vi "rsidr_core_global.vi"() -> ()   [LabVIEW 2015, in "Rohde&Schwarz CMXP NR FR2 Measurement.lvlib"] (continued)
peak values for low and high EVM window position, for all measured list mode segments.\n\nAvailable Repeated Capabilities:\ninstance: i0, i1, i2, i3, i4, i5, i6, i7, i8, i9, i10, i11, i12, i13, i14, i15, i16, i17, i18, i19, i20, i21, i22, i23, i24, i25, i26, i27, i28, i29, i30, i31, i32\r\n\nRemote-control command(s):\nCALCulate:NRMMw:MEAS<i>:MEValuation:LIST:MODulation:PERRor:PEAK:LOW:CURRent?"}, {"Level"=5, "Class Only"=FALSE, "Identifier"="RSCMXPNRFR2M_ATTR_QUERY_MULTI_EVAL_MEASUREMENT_LIST_PERR_PEAK_LOW_EXTREME_LIMIT_CHECK_RESULTS", "Descriptive Name"="Query Multi Eval Measurement List PERR Peak Low Extreme Limit Check Results", "Data Type"=enum."RawString", "Command"="CALC:NRMM:MEAS{instance}:MEV:LIST:MOD:PERR:PEAK:LOW:EXTR?", "Access"=enum."Read Only", "Range Table"="", "Read Callback"="", "Write Callback"="", "Range Callback"="", "Check Callback"="", "Rngtable Callback"="", "Coerce Callback"="", "Supported Models"="", "Instrument Options"="", "Check Status Callback"="", "Flags"=0, "Help"="Returns the limit check results for the phase error peak values for low and high EVM window position, for all measured list mode segments.\n\nAvailable Repeated Capabilities:\ninstance: i0, i1, i2, i3, i4, i5, i6, i7, i8, i9, i10, i11, i12, i13, i14, i15, i16, i17, i18, i19, i20, i21, i22, i23, i24, i25, i26, i27, i28, i29, i30, i31, i32\r\n\nRemote-control command(s):\nCALCulate:NRMMw:MEAS<i>:MEValuation:LIST:MODulation:PERRor:PEAK:LOW:EXTReme?"}, {"Level"=5, "Class Only"=FALSE, "Identifier"="RSCMXPNRFR2M_ATTR_FETCH_MULTI_EVAL_MEASUREMENT_LIST_PERR_RMS_HIGH_AVERAGE_RESULTS", "Descriptive Name"="Fetch Multi Eval Measurement List PERR RMS High Average Results", "Data Type"=enum."RawString", "Command"="FETC:NRMM:MEAS{instance}:MEV:LIST:MOD:PERR:RMS:HIGH:AVER?", "Access"=enum."Read Only", "Range Table"="", "Read Callback"="", "Write Callback"="", "Range Callback"="", "Check Callback"="", "Rngtable Callback"="", "Coerce Callback"="", "Supported Models"="", "Instrument Options"="", "Check Status Callback"="", "Flags"=0, "Help"="Returns phase error RMS values for low and high EVM window position, for all measured list mode segments.\n\nAvailable Repeated Capabilities:\ninstance: i0, i1, i2, i3, i4, i5, i6, i7, i8, i9, i10, i11, i12, i13, i14, i15, i16, i17, i18, i19, i20, i21, i22, i23, i24, i25, i26, i27, i28, i29, i30, i31, i32\r\n\nRemote-control command(s):\nFETCh:NRMMw:MEAS<i>:MEValuation:LIST:MODulation:PERRor:RMS:HIGH:AVERage?"}, {"Level"=5, "Class Only"=FALSE, "Identifier"="RSCMXPNRFR2M_ATTR_FETCH_MULTI_EVAL_MEASUREMENT_LIST_PERR_RMS_HIGH_CURRENT_RESULTS", "Descriptive Name"="Fetch Multi Eval Measurement List PERR RMS High Current Results", "Data Type"=enum."RawString", "Command"="FETC:NRMM:MEAS{instance}:MEV:LIST:MOD:PERR:RMS:HIGH:CURR?", "Access"=enum."Read Only", "Range Table"="", "Read Callback"="", "Write Callback"="", "Range Callback"="", "Check Callback"="", "Rngtable Callback"="", "Coerce Callback"="", "Supported Models"="", "Instrument Options"="", "Check Status Callback"="", "Flags"=0, "Help"="Returns phase error RMS values for low and high EVM window position, for all measured list mode segments.\n\nAvailable Repeated Capabilities:\ninstance: i0, i1, i2, i3, i4, i5, i6, i7, i8, i9, i10, i11, i12, i13, i14, i15, i16, i17, i18, i19, i20, i21, i22, i23, i24, i25, i26, i27, i28, i29, i30, i31, i32\r\n\nRemote-control command(s):\nFETCh:NRMMw:MEAS<i>:MEValuation:LIST:MODulation:PERRor:RMS:HIGH:CURRent?"}, {"Level"=5, "Class Only"=FALSE, "Identifier"="RSCMXPNRFR2M_ATTR_FETCH_MULTI_EVAL_MEASUREMENT_LIST_PERR_RMS_HIGH_EXTREME_RESULTS", "Descriptive Name"="Fetch Multi Eval Measurement List PERR RMS High Extreme Results", "Data Type"=enum."RawString", "Command"="FETC:NRMM:MEAS{instance}:MEV:LIST:MOD:PERR:RMS:HIGH:EXTR?", "Access"=enum."Read Only", "Range Table"="", "Read Callback"="", "Write Callback"="", "Range Callback"="", "Check Callback"="", "Rngtable Callback"="", "Coerce Callback"="", "Supported Models"="", "Instrument Options"="", "Check Status Callback"="", "Flags"=0, "Help"="Returns phase error RMS values for low and high EVM window position, for all measured list mode segments.\n\nAvailable Repeated Capabilities:\ninstance: i0, i1, i2, i3, i4, i5, i6, i7, i8, i9, i10, i11, i12, i13, i14, i15, i16, i17, i18, i19, i20, i21, i22, i23, i24, i25, i26, i27, i28, i29, i30, i31, i32\r\n\nRemote-control command(s):\nFETCh:NRMMw:MEAS<i>:MEValuation:LIST:MODulation:PERRor:RMS:HIGH:EXTReme?"}, {"Level"=5, "Class Only"=FALSE, "Identifier"="RSCMXPNRFR2M_ATTR_FETCH_MULTI_EVAL_MEASUREMENT_LIST_PERR_RMS_HIGH_STANDARD_DEVIATION_RESULTS", "Descriptive Name"="Fetch Multi Eval Measurement List PERR RMS High Standard Deviation Results", "Data Type"=enum."RawString", "Command"="FETC:NRMM:MEAS{instance}:MEV:LIST:MOD:PERR:RMS:HIGH:SDEV?", "Access"=enum."Read Only", "Range Table"="", "Read Callback"="", "Write Callback"="", "Range Callback"="", "Check Callback"="", "Rngtable Callback"="", "Coerce Callback"="", "Supported Models"="", "Instrument Options"="", "Check Status Callback"="", "Flags"=0, "Help"="Returns phase error RMS values for low and high EVM window position, for all measured list mode segments.\n\nAvailable Repeated Capabilities:\ninstance: i0, i1, i2, i3, i4, i5, i6, i7, i8, i9, i10, i11, i12, i13, i14, i15, i16, i17, i18, i19, i20, i21, i22, i23, i24, i25, i26, i27, i28, i29, i30, i31, i32\r\n\nRemote-control command(s):\nFETCh:NRMMw:MEAS<i>:MEValuation:LIST:MODulation:PERRor:RMS:HIGH:SDEViation?"}, {"Level"=5, "Class Only"=FALSE, "Identifier"="RSCMXPNRFR2M_ATTR_FETCH_MULTI_EVAL_MEASUREMENT_LIST_PERR_RMS_LOW_AVERAGE_RESULTS", "Descriptive Name"="Fetch Multi Eval Measurement List PERR RMS Low Average Results", "Data Type"=enum."RawString", "Command"="FETC:NRMM:MEAS{instance}:MEV:LIST:MOD:PERR:RMS:LOW:AVER?", "Access"=enum."Read Only", "Range Table"="", "Read Callback"="", "Write Callback"="", "Range Callback"="", "Check Callback"="", "Rngtable Callback"="", "Coerce Callback"="", "Supported Models"="", "Instrument Options"="", "Check Status Callback"="", "Flags"=0, "Help"="Returns phase error RMS values for low and high EVM window position, for all measured list mode segments.\n\nAvailable Repeated Capabilities:\ninstance: i0, i1, i2, i3, i4, i5, i6, i7, i8, i9, i10, i11, i12, i13, i14, i15, i16, i17, i18, i19, i20, i21, i22, i23, i24, i25, i26, i27, i28, i29, i30, i31, i32\r\n\nRemote-control command(s):\nFETCh:NRMMw:MEAS<i>:MEValuation:LIST:MODulation:PERRor:RMS:LOW:AVERage?"}, {"Level"=5, "Class Only"=FALSE, "Identifier"="RSCMXPNRFR2M_ATTR_FETCH_MULTI_EVAL_MEASUREMENT_LIST_PERR_RMS_LOW_CURRENT_RESULTS", "Descriptive Name"="Fetch Multi Eval Measurement List PERR RMS Low Current Results", "Data Type"=enum."RawString", "Command"="FETC:NRMM:MEAS{instance}:MEV:LIST:MOD:PERR:RMS:LOW:CURR?", "Access"=enum."Read Only", "Range Table"="", "Read Callback"="", "Write Callback"="", "Range Callback"="", "Check Callback"="", "Rngtable Callback"="", "Coerce Callback"="", "Supported Models"="", "Instrument Options"="", "Check Status Callback"="", "Flags"=0, "Help"="Returns phase error RMS values for low and high EVM window position, for all measured list mode segments.\n\nAvailable Repeated Capabilities:\ninstance: i0, i1, i2, i3, i4, i5, i6, i7, i8, i9, i10, i11, i12, i13, i14, i15, i16, i17, i18, i19, i20, i21, i22, i23, i24, i25, i26, i27, i28, i29, i30, i31, i32\r\n\nRemote-control command(s):\nFETCh:NRMMw:MEAS<i>:MEValuation:LIST:MODulation:PERRor:RMS:LOW:CURRent?"}, {"Level"=5, "Class Only"=FALSE, "Identifier"="RSCMXPNRFR2M_ATTR_FETCH_MULTI_EVAL_MEASUREMENT_LIST_PERR_RMS_LOW_EXTREME_RESULTS", "Descriptive Name"="Fetch Multi Eval Measurement List PERR RMS Low Extreme Results", "Data Type"=enum."RawString", "Command"="FETC:NRMM:MEAS{instance}:MEV:LIST:MOD:PERR:RMS:LOW:EXTR?", "Access"=enum."Read Only", "Range Table"="", "Read Callback"="", "Write Callback"="", "Range Callback"="", "Check Callback"="", "Rngtable Callback"="", "Coerce Callback"="", "Supported Models"="", "Instrument Options"="", "Check Status Callback"="", "Flags"=0, "Help"="Returns phase error RMS values for low and high EVM window position, for all measured list mode segments.\n\nAvailable Repeated Capabilities:\ninstance: i0, i1, i2, i3, i4, i5, i6, i7, i8, i9, i10, i11, i12, i13, i14, i15, i16, i17, i18, i19, i20, i21, i22, i23, i24, i25, i26, i27, i28, i29, i30, i31, i32\r\n\nRemote-control command(s):\nFETCh:NRMMw:MEAS<i>:MEValuation:LIST:MODulation:PERRor:RMS:LOW:EXTReme?"}, {"Level"=5, "Class Only"=FALSE, "Identifier"="RSCMXPNRFR2M_ATTR_FETCH_MULTI_EVAL_MEASUREMENT_LIST_PERR_RMS_LOW_STANDARD_DEVIATION_RESULTS", "Descriptive Name"="Fetch Multi Eval Measurement List PERR RMS Low Standard Deviation Results", "Data Type"=enum."RawString", "Command"="FETC:NRMM:MEAS{instance}:MEV:LIST:MOD:PERR:RMS:LOW:SDEV?", "Access"=enum."Read Only", "Range Table"="", "Read Callback"="", "Write Callback"="", "Range Callback"="", "Check Callback"="", "Rngtable Callback"="", "Coerce Callback"="", "Supported Models"="", "Instrument Options"="", "Check Status Callback"="", "Flags"=0, "Help"="Returns phase error RMS values for low and high EVM window position, for all measured list mode segments.\n\nAvailable Repeated Capabilities:\ninstance: i0, i1, i2, i3, i4, i5, i6, i7, i8, i9, i10, i11, i12, i13, i14, i15, i16, i17, i18, i19, i20, i21, i22, i23, i24, i25, i26, i27, i28, i29, i30, i31, i32\r\n\nRemote-control command(s):\nFETCh:NRMMw:MEAS<i>:MEValuation:LIST:MODulation:PERRor:RMS:LOW:SDEViation?"}, {"Level"=5, "Class Only"=FALSE, "Identifier"="RSCMXPNRFR2M_ATTR_QUERY_MULTI_EVAL_MEASUREMENT_LIST_PERR_RMS_HIGH_AVERAGE_LIMIT_CHECK_RESULTS", "Descriptive Name"="Query Multi Eval Measurement List PERR RMS High Average Limit Check Results", "Data Type"=enum."RawString", "Command"="CALC:NRMM:MEAS{instance}:MEV:LIST:MOD:PERR:RMS:HIGH:AVER?", "Access"=enum."Read Only", "Range Table"="", "Read Callback"="", "Write Callback"="", "Range Callback"="", "Check Callback"="", "Rngtable Callback"="", "Coerce Callback"="", "Supported Models"="", "Instrument Options"="", "Check Status Callback"="", "Flags"=0, "Help"="Returns the limit check results for the phase error RMS values for low and high EVM window position, for all measured list mode segments.\n\nAvailable Repeated Capabilities:\ninstance: i0, i1, i2, i3, i4, i5, i6, i7, i8, i9, i10, i11, i12, i13, i14, i15, i16, i17, i18, i19, i20, i21, i22, i23, i24, i25, i26, i27, i28, i29, i30, i31, i32\r\n\nRemote-control command(s):\nCALCulate:NRMMw:MEAS<i>:MEValuation:LIST:MODulation:PERRor:RMS:HIGH:AVERage?"}, {"Level"=5, "Class Only"=FALSE, "Identifier"="RSCMXPNRFR2M_ATTR_QUERY_MULTI_EVAL_MEASUREMENT_LIST_PERR_RMS_HIGH_CURRENT_LIMIT_CHECK_RESULTS", "Descriptive Name"="Query Multi Eval Measurement List PERR RMS High Current Limit Check Results", "Data Type"=enum."RawString", "Command"="CALC:NRMM:MEAS{instance}:MEV:LIST:MOD:PERR:RMS:HIGH:CURR?", "Access"=enum."Read Only", "Range Table"="", "Read Callback"="", "Write Callback"="", "Range Callback"="", "Check Callback"="", "Rngtable Callback"="", "Coerce Callback"="", "Supported Models"="", "Instrument Options"="", "Check Status Callback"="", "Flags"=0, "Help"="Returns the limit check results for the phase error RMS values for low and high EVM window position, for all measured list mode segments.\n\nAvailable Repeated Capabilities:\ninstance: i0, i1, i2, i3, i4, i5, i6, i7, i8, i9, i10, i11, i12, i13, i14, i15, i16, i17, i18, i19, i20, i21, i22, i23, i24, i25, i26, i27, i28, i29, i30, i31, i32\r\n\nRemote-control command(s):\nCALCulate:NRMMw:MEAS<i>:MEValuation:LIST:MODulation:PERRor:RMS:HIGH:CURRent?"}, {"Level"=5, "Class Only"=FALSE, "Identifier"="RSCMXPNRFR2M_ATTR_QUERY_MULTI_EVAL_MEASUREMENT_LIST_PERR_RMS_HIGH_EXTREME_LIMIT_CHECK_RESULTS", "Descriptive Name"="Query Multi Eval Measurement List PERR RMS High Extreme Limit Check Results", "Data Type"=enum."RawString", "Command"="CALC:NRMM:MEAS{instance}:MEV:LIST:MOD:PERR:RMS:HIGH:EXTR?", "Access"=enum."Read Only", "Range Table"="", "Read Callback"="", "Write Callback"="", "Range Callback"="", "Check Callback"="", "Rngtable Callback"="", "Coerce Callback"="", "Supported Models"="", "Instrument Options"="", "Check Status Callback"="", "Flags"=0, "Help"="Returns the limit check results for the phase error RMS values for low and high EVM window position, for all measured list mode segments.\n\nAvailable Repeated Capabilities:\ninstance: i0, i1, i2, i3, i4, i5, i6, i7, i8, i9, i10, i11, i12, i13, i14, i15, i16, i17, i18, i19, i20, i21, i22, i23, i24, i25, i26, i27, i28, i29, i30, i31, i32\r\n\nRemote-control command(s):\nCALCulate:NRMMw:MEAS<i>:MEValuation:LIST:MODulation:PERRor:RMS:HIGH:EXTReme?"}, {"Level"=5, "Class Only"=FALSE, "Identifier"="RSCMXPNRFR2M_ATTR_QUERY_MULTI_EVAL_MEASUREMENT_LIST_PERR_RMS_LOW_AVERAGE_LIMIT_CHECK_RESULTS", "Descriptive Name"="Query Multi Eval Measurement List PERR RMS Low Average Limit Check Results", "Data Type"=enum."RawString", "Command"="CALC:NRMM:MEAS{instance}:MEV:LIST:MOD:PERR:RMS:LOW:AVER?", "Access"=enum."Read Only", "Range Table"="", "Read Callback"="", "Write Callback"="", "Range Callback"="", "Check Callback"="", "Rngtable Callback"="", "Coerce Callback"="", "Supported Models"="", "Instrument Options"="", "Check Status Callback"="", "Flags"=0, "Help"="Returns the limit check results for the phase error RMS values for low and high EVM window position, for all measured list mode segments.\n\nAvailable Repeated Capabilities:\ninstance: i0, i1, i2, i3, i4, i5, i6, i7, i8, i9, i10, i11, i12, i13, i14, i15, i16, i17, i18, i19, i20, i21, i22, i23, i24, i25, i26, i27, i28, i29, i30, i31, i32\r\n\nRemote-control command(s):\nCALCulate:NRMMw:MEAS<i>:MEValuation:LIST:MODulation:PERRor:RMS:LOW:AVERage?"}, {"Level"=5, "Class Only"=FALSE, "Identifier"="RSCMXPNRFR2M_ATTR_QUERY_MULTI_EVAL_MEASUREMENT_LIST_PERR_RMS_LOW_CURRENT_LIMIT_CHECK_RESULTS", "Descriptive Name"="Query Multi Eval Measurement List PERR RMS Low Current Limit Check Results", "Data Type"=enum."RawString", "Command"="CALC:NRMM:MEAS{instance}:MEV:LIST:MOD:PERR:RMS:LOW:CURR?", "Access"=enum."Read Only", "Range Table"="", "Read Callback"="", "Write Callback"="", "Range Callback"="", "Check Callback"="", "Rngtable Callback"="", "Coerce Callback"="", "Supported Models"="", "Instrument Options"="", "Check Status Callback"="", "Flags"=0, "Help"="Returns the limit check results for the phase error RMS values for low and high EVM window position, for all measured list mode segments.\n\nAvailable Repeated Capabilities:\ninstance: i0, i1, i2, i3, i4, i5, i6, i7, i8, i9, i10, i11, i12, i13, i14, i15, i16, i17, i18, i19, i20, i21, i22, i23, i24, i25, i26, i27, i28, i29, i30, i31, i32\r\n\nRemote-control command(s):\nCALCulate:NRMMw:MEAS<i>:MEValuation:LIST:MODulation:PERRor:RMS:LOW:CURRent?"}, {"Level"=5, "Class Only"=FALSE, "Identifier"="RSCMXPNRFR2M_ATTR_QUERY_MULTI_EVAL_MEASUREMENT_LIST_PERR_RMS_LOW_EXTREME_LIMIT_CHECK_RESULTS", "Descriptive Name"="Query Multi Eval Measurement List PERR RMS Low Extreme Limit Check Results", "Data Type"=enum."RawString", "Command"="CALC:NRMM:MEAS{instance}:MEV:LIST:MOD:PERR:RMS:LOW:EXTR?", "Access"=enum."Read Only", "Range Table"="", "Read Callback"="", "Write Callback"="", "Range Callback"="", "Check Callback"="", "Rngtable Callback"="", "Coerce Callback"="", "Supported Models"="", "Instrument Options"="", "Check Status Callback"="", "Flags"=0, "Help"="Returns the limit check results for the phase error RMS values for low and high EVM window position, for all measured list mode segments.\n\nAvailable Repeated Capabilities:\ninstance: i0, i1, i2, i3, i4, i5, i6, i7, i8, i9, i10, i11, i12, i13, i14, i15, i16, i17, i18, i19, i20, i21, i22, i23, i24, i25, i26, i27, i28, i29, i30, i31, i32\r\n\nRemote-control command(s):\nCALCulate:NRMMw:MEAS<i>:MEValuation:LIST:MODulation:PERRor:RMS:LOW:EXTReme?"}, {"Level"=4, "Class Only"=TRUE, "Identifier"="", "Descriptive Name"="Peak Power", "Data Type"=enum."ViInt32", "Command"="", "Access"=enum."Read Only", "Range Table"="", "Read Callback"="", "Write Callback"="", "Range Callback"="", "Check Callback"="", "Rngtable Callback"="", "Coerce Callback"="", "Supported Models"="", "Instrument Options"="", "Check Status Callback"="", "Flags"=0, "Help"="The following attributes return user equipment peak power values for all measured list mode segments."}, {"Level"=5, "Class Only"=FALSE, "Identifier"="RSCMXPNRFR2M_ATTR_FETCH_MULTI_EVAL_MEASUREMENT_LIST_PEAK_POWER_AVERAGE_RESULTS", "Descriptive Name"="Fetch Multi Eval Measurement List Peak Power Average Results", "Data Type"=enum."RawString", "Command"="FETC:NRMM:MEAS{instance}:MEV:LIST:MOD:PPOW:AVER?", "Access"=enum."Read Only", "Range Table"="", "Read Callback"="", "Write Callback"="", "Range Callback"="", "Check Callback"="", "Rngtable Callback"="", "Coerce Callback"="", "Supported Models"="", "Instrument Options"="", "Check Status Callback"="", "Flags"=0, "Help"="Returns user equipment peak power values for all measured list mode segments.\n\nAvailable Repeated Capabilities:\ninstance: i0, i1, i2, i3, i4, i5, i6, i7, i8, i9, i10, i11, i12, i13, i14, i15, i16, i17, i18, i19, i20, i21, i22, i23, i24, i25, i26, i27, i28, i29, i30, i31, i32\r\n\nRemote-control command(s):\nFETCh:NRMMw:MEAS<i>:MEValuation:LIST:MODulation:PPOWer:AVERage?"}, {"Level"=5, "Class Only"=FALSE, "Identifier"="RSCMXPNRFR2M_ATTR_FETCH_MULTI_EVAL_MEASUREMENT_LIST_PEAK_POWER_CURRENT_RESULTS", "Descriptive Name"="Fetch Multi Eval Measurement List Peak Power Current Results", "Data Type"=enum."RawString", "Command"="FETC:NRMM:MEAS{instance}:MEV:LIST:MOD:PPOW:CURR?", "Access"=enum."Read Only", "Range Table"="", "Read Callback"="", "Write Callback"="", "Range Callback"="", "Check Callback"="", "Rngtable Callback"="", "Coerce Callback"="", "Supported Models"="", "Instrument Options"="", "Check Status Callback"="", "Flags"=0, "Help"="Returns user equipment peak power values for all measured list mode segments.\n\nAvailable Repeated Capabilities:\ninstance: i0, i1, i2, i3, i4, i5, i6, i7, i8, i9, i10, i11, i12, i13, i14, i15, i16, i17, i18, i19, i20, i21, i22, i23, i24, i25, i26, i27, i28, i29, i30, i31, i32\r\n\nRemote-control command(s):\nFETCh:NRMMw:MEAS<i>:MEValuation:LIST:MODulation:PPOWer:CURRent?"}, {"Level"=5, "Class Only"=FALSE, "Identifier"="RSCMXPNRFR2M_ATTR_FETCH_MULTI_EVAL_MEASUREMENT_LIST_PEAK_POWER_MAXIMUM_RESULTS", "Descriptive Name"="Fetch Multi Eval Measurement List Peak Power Maximum Results", "Data Type"=enum."RawString", "Command"="FETC:NRMM:MEAS{instance}:MEV:LIST:MOD:PPOW:MAX?", "Access"=enum."Read Only", "Range Table"="", "Read Callback"="", "Write Callback"="", "Range Callback"="", "Check Callback"="", "Rngtable Callback"="", "Coerce Callback"="", "Supported Models"="", "Instrument Options"="", "Check Status Callback"="", "Flags"=0, "Help"="Returns user equipment peak power values for all measured list mode segments.\n\nAvailable Repeated Capabilities:\ninstance: i0, i1, i2, i3, i4, i5, i6, i7, i8, i9, i10, i11, i12, i13, i14, i15, i16, i17, i18, i19, i20, i21, i22, i23, i24, i25, i26, i27, i28, i29, i30, i31, i32\r\n\nRemote-control command(s):\nFETCh:NRMMw:MEAS<i>:MEValuation:LIST:MODulation:PPOWer:MAXimum?"}, {"Level"=5, "Class Only"=FALSE, "Identifier"="RSCMXPNRFR2M_ATTR_FETCH_MULTI_EVAL_MEASUREMENT_LIST_PEAK_POWER_MINIMUM_RESULTS", "Descriptive Name"="Fetch Multi Eval Measurement List Peak Power Minimum Results", "Data Type"=enum."RawString", "Command"="FETC:NRMM:MEAS{instance}:MEV:LIST:MOD:PPOW:MIN?", "Access"=enum."Read Only", "Range Table"="", "Read Callback"="", "Write Callback"="", "Range Callback"="", "Check Callback"="", "Rngtable Callback"="", "Coerce Callback"="", "Supported Models"="", "Instrument Options"="", "Check Status Callback"="", "Flags"=0, "Help"="Returns user equipment peak power values for all measured list mode segments.\n\nAvailable Repeated Capabilities:\ninstance: i0, i1, i2, i3, i4, i5, i6, i7, i8, i9, i10, i11, i12, i13, i14, i15, i16, i17, i18, i19, i20, i21, i22, i23, i24, i25, i26, i27, i28, i29, i30, i31, i32\r\n\nRemote-control command(s):\nFETCh:NRMMw:MEAS<i>:MEValuation:LIST:MODulation:PPOWer:MINimum?"}, {"Level"=5, "Class Only"=FALSE, "Identifier"="RSCMXPNRFR2M_ATTR_FETCH_MULTI_EVAL_MEASUREMENT_LIST_PEAK_POWER_STANDARD_DEVIATION_RESULTS", "Descriptive Name"="Fetch Multi Eval Measurement List Peak Power Standard Deviation Results", "Data Type"=enum."RawString", "Command"="FETC:NRMM:MEAS{instance}:MEV:LIST:MOD:PPOW:SDEV?", "Access"=enum."Read Only", "Range Table"="", "Read Callback"="", "Write Callback"="", "Range Callback"="", "Check Callback"="", "Rngtable Callback"="", "Coerce Callback"="", "Supported Models"="", "Instrument Options"="", "Check Status Callback"="", "Flags"=0, "Help"="Returns user equipment peak power values for all measured list mode segments.\n\nAvailable Repeated Capabilities:\ninstance: i0, i1, i2, i3, i4, i5, i6, i7, i8, i9, i10, i11, i12, i13, i14, i15, i16, i17, i18, i19, i20, i21, i22, i23, i24, i25, i26, i27, i28, i29, i30, i31, i32\r\n\nRemote-control command(s):\nFETCh:NRMMw:MEAS<i>:MEValuation:LIST:MODulation:PPOWer:SDEViation?"}, {"Level"=5, "Class Only"=FALSE, "Identifier"="RSCMXPNRFR2M_ATTR_QUERY_MULTI_EVAL_MEASUREMENT_LIST_PEAK_POWER_AVERAGE_LIMIT_CHECK_RESULTS", "Descriptive Name"="Query Multi Eval Measurement List Peak Power Average Limit Check Results", "Data Type"=enum."RawString", "Command"="CALC:NRMM:MEAS{instance}:MEV:LIST:MOD:PPOW:AVER?", "Access"=enum."Read Only", "Range Table"="", "Read Callback"="", "Write Callback"="", "Range Callback"="", "Check Callback"="", "Rngtable Callback"="", "Coerce Callback"="", "Supported Models"="", "Instrument Options"="", "Check Status Callback"="", "Flags"=0, "Help"="Returns the limit check results for the user equipment peak power values for all measured list mode segments.\n\nAvailable Repeated Capabilities:\ninstance: i0, i1, i2, i3, i4, i5, i6, i7, i8, i9, i10, i11, i12, i13, i14, i15, i16, i17, i18, i19, i20, i21, i22, i23, i24, i25, i26, i27, i28, i29, i30, i31, i32\r\n\nRemote-control command(s):\nCALCulate:NRMMw:MEAS<i>:MEValuation:LIST:MODulation:PPOWer:AVERage?"}, {"Level"=5, "Class Only"=FALSE, "Identifier"="RSCMXPNRFR2M_ATTR_QUERY_MULTI_EVAL_MEASUREMENT_LIST_PEAK_POWER_CURRENT_LIMIT_CHECK_RESULTS", "Descriptive Name"="Query Multi Eval Measurement List Peak Power Current Limit Check Results", "Data Type"=enum."RawString", "Command"="CALC:NRMM:MEAS{instance}:MEV:LIST:MOD:PPOW:CURR?", "Access"=enum."Read Only", "Range Table"="", "Read Callback"="", "Write Callback"="", "Range Callback"="", "Check Callback"="", "Rngtable Callback"="", "Coerce Callback"="", "Supported Models"="", "Instrument Options"="", "Check Status Callback"="", "Flags"=0, "Help"="Returns the limit check results for the user equipment peak power values for all measured list mode segments.\n\nAvailable Repeated Capabilities:\ninstance: i0, i1, i2, i3, i4, i5, i6, i7, i8, i9, i10, i11, i12, i13, i14, i15, i16, i17, i18, i19, i20, i21, i22, i23, i24, i25, i26, i27, i28, i29, i30, i31, i32\r\n\nRemote-control command(s):\nCALCulate:NRMMw:MEAS<i>:MEValuation:LIST:MODulation:PPOWer:CURRent?"}, {"Level"=5, "Class Only"=FALSE, "Identifier"="RSCMXPNRFR2M_ATTR_QUERY_MULTI_EVAL_MEASUREMENT_LIST_PEAK_POWER_MAXIMUM_LIMIT_CHECK_RESULTS", "Descriptive Name"="Query Multi Eval Measurement List Peak Power Maximum Limit Check Results", "Data Type"=enum."RawString", "Command"="CALC:NRMM:MEAS{instance}:MEV:LIST:MOD:PPOW:MAX?", "Access"=enum."Read Only", "Range Table"="", "Read Callback"="", "Write Callback"="", "Range Callback"="", "Check Callback"="", "Rngtable Callback"="", "Coerce Callback"="", "Supported Models"="", "Instrument Options"="", "Check Status Callback"="", "Flags"=0, "Help"="Returns the limit check results for the user equipment peak power values for all measured list mode segments.\n\nAvailable Repeated Capabilities:\ninstance: i0, i1, i2, i3, i4, i5, i6, i7, i8, i9, i10, i11, i12, i13, i14, i15, i16, i17, i18, i19, i20, i21, i22, i23, i24, i25, i26, i27, i28, i29, i30, i31, i32\r\n\nRemote-control command(s):\nCALCulate:NRMMw:MEAS<i>:MEValuation:LIST:MODulation:PPOWer:MAXimum?"}, {"Level"=5, "Class Only"=FALSE, "Identifier"="RSCMXPNRFR2M_ATTR_QUERY_MULTI_EVAL_MEASUREMENT_LIST_PEAK_POWER_MINIMUM_LIMIT_CHECK_RESULTS", "Descriptive Name"="Query Multi Eval Measurement List Peak Power Minimum Limit Check Results", "Data Type"=enum."RawString", "Command"="CALC:NRMM:MEAS{instance}:MEV:LIST:MOD:PPOW:MIN?", "Access"=enum."Read Only", "Range Table"="", "Read Callback"="", "Write Callback"="", "Range Callback"="", "Check Callback"="", "Rngtable Callback"="", "Coerce Callback"="", "Supported Models"="", "Instrument Options"="", "Check Status Callback"="", "Flags"=0, "Help"="Returns the limit check results for the user equipment peak power values for all measured list mode segments.\n\nAvailable Repeated Capabilities:\ninstance: i0, i1, i2, i3, i4, i5, i6, i7, i8, i9, i10, i11, i12, i13, i14, i15, i16, i17, i18, i19, i20, i21, i22, i23, i24, i25, i26, i27, i28, i29, i30, i31, i32\r\n\nRemote-control command(s):\nCALCulate:NRMMw:MEAS<i>:MEValuation:LIST:MODulation:PPOWer:MINimum?"}, {"Level"=4, "Class Only"=TRUE, "Identifier"="", "Descriptive Name"="Power Spectral Density", "Data Type"=enum."ViInt32", "Command"="", "Access"=enum."Read Only", "Range Table"="", "Read Callback"="", "Write Callback"="", "Range Callback"="", "Check Callback"="", "Rngtable Callback"="", "Coerce Callback"="", "Supported Models"="", "Instrument Options"="", "Check Status Callback"="", "Flags"=0, "Help"="The following attributes return RB power values (power spectral density) for all measured list mode segments."}, {"Level"=5, "Class Only"=FALSE, "Identifier"="RSCMXPNRFR2M_ATTR_FETCH_MULTI_EVAL_MEASUREMENT_LIST_POWER_SPECTRAL_DENSITY_AVERAGE_RESULTS", "Descriptive Name"="Fetch Multi Eval Measurement List Power Spectral Density Average Results", "Data Type"=enum."RawString", "Command"="FETC:NRMM:MEAS{instance}:MEV:LIST:MOD:PSD:AVER?", "Access"=enum."Read Only", "Range Table"="", "Read Callback"="", "Write Callback"="", "Range Callback"="", "Check Callback"="", "Rngtable Callback"="", "Coerce Callback"="", "Supported Models"="", "Instrument Options"="", "Check Status Callback"="", "Flags"=0, "Help"="Returns RB power values (power spectral density) for all measured list mode segments.\n\nAvailable Repeated Capabilities:\ninstance: i0, i1, i2, i3, i4, i5, i6, i7, i8, i9, i10, i11, i12, i13, i14, i15, i16, i17, i18, i19, i20, i21, i22, i23, i24, i25, i26, i27, i28, i29, i30, i31, i32\r\n\nRemote-control command(s):\nFETCh:NRMMw:MEAS<i>:MEValuation:LIST:MODulation:PSD:AVERage?"}, {"Level"=5, "Class Only"=FALSE, "Identifier"="RSCMXPNRFR2M_ATTR_FETCH_MULTI_EVAL_MEASUREMENT_LIST_POWER_SPECTRAL_DENSITY_CURRENT_RESULTS", "Descriptive Name"="Fetch Multi Eval Measurement List Power Spectral Density Current Results", "Data Type"=enum."RawString", "Command"="FETC:NRMM:MEAS{instance}:MEV:LIST:MOD:PSD:CURR?", "Access"=enum."Read Only", "Range Table"="", "Read Callback"="", "Write Callback"="", "Range Callback"="", "Check Callback"="", "Rngtable Callback"="", "Coerce Callback"="", "Supported Models"="", "Instrument Options"="", "Check Status Callback"="", "Flags"=0, "Help"="Returns RB power values (power spectral density) for all measured list mode segments.\n\nAvailable Repeated Capabilities:\ninstance: i0, i1, i2, i3, i4, i5, i6, i7, i8, i9, i10, i11, i12, i13, i14, i15, i16, i17, i18, i19, i20, i21, i22, i23, i24, i25, i26, i27, i28, i29, i30, i31, i32\r\n\nRemote-control command(s):\nFETCh:NRMMw:MEAS<i>:MEValuation:LIST:MODulation:PSD:CURRent?"}, {"Level"=5, "Class Only"=FALSE, "Identifier"="RSCMXPNRFR2M_ATTR_FETCH_MULTI_EVAL_MEASUREMENT_LIST_POWER_SPECTRAL_DENSITY_MAXIMUM_RESULTS", "Descriptive Name"="Fetch Multi Eval Measurement List Power Spectral Density Maximum Results", "Data Type"=enum."RawString", "Command"="FETC:NRMM:MEAS{instance}:MEV:LIST:MOD:PSD:MAX?", "Access"=enum."Read Only", "Range Table"="", "Read Callback"="", "Write Callback"="", "Range Callback"="", "Check Callback"="", "Rngtable Callback"="", "Coerce Callback"="", "Supported Models"="", "Instrument Options"="", "Check Status Callback"="", "Flags"=0, "Help"="Returns RB power values (power spectral density) for all measured list mode segments.\n\nAvailable Repeated Capabilities:\ninstance: i0, i1, i2, i3, i4, i5, i6, i7, i8, i9, i10, i11, i12, i13, i14, i15, i16, i17, i18, i19, i20, i21, i22, i23, i24, i25, i26, i27, i28, i29, i30, i31, i32\r\n\nRemote-control command(s):\nFETCh:NRMMw:MEAS<i>:MEValuation:LIST:MODulation:PSD:MAXimum?"}, {"Level"=5, "Class Only"=FALSE, "Identifier"="RSCMXPNRFR2M_ATTR_FETCH_MULTI_EVAL_MEASUREMENT_LIST_POWER_SPECTRAL_DENSITY_MINIMUM_RESULTS", "Descriptive Name"="Fetch Multi Eval Measurement List Power Spectral Density Minimum Results", "Data Type"=enum."RawString", "Command"="FETC:NRMM:MEAS{instance}:MEV:LIST:MOD:PSD:MIN?", "Access"=enum."Read Only", "Range Table"="", "Read Callback"="", "Write Callback"="", "Range Callback"="", "Check Callback"="", "Rngtable Callback"="", "Coerce Callback"="", "Supported Models"="", "Instrument Options"="", "Check Status Callback"="", "Flags"=0, "Help"="Returns RB power values (power spectral density) for all measured list mode segments.\n\nAvailable Repeated Capabilities:\ninstance: i0, i1, i2, i3, i4, i5, i6, i7, i8, i9, i10, i11, i12, i13, i14, i15, i16, i17, i18, i19, i20, i21, i22, i23, i24, i25, i26, i27, i28, i29, i30, i31, i32\r\n\nRemote-control command(s):\nFETCh:NRMMw:MEAS<i>:MEValuation:LIST:MODulation:PSD:MINimum?"}, {"Level"=5, "Class Only"=FALSE, "Identifier"="RSCMXPNRFR2M_ATTR_FETCH_MULTI_EVAL_MEASUREMENT_LIST_POWER_SPECTRAL_DENSITY_STANDARD_DEVIATION_RESULTS", "Descriptive Name"="Fetch Multi Eval Measurement List Power Spectral Density Standard Deviation Results", "Data Type"=enum."RawString", "Command"="FETC:NRMM:MEAS{instance}:MEV:LIST:MOD:PSD:SDEV?", "Access"=enum."Read Only", "Range Table"="", "Read Callback"="", "Write Callback"="", "Range Callback"="", "Check Callback"="", "Rngtable Callback"="", "Coerce Callback"="", "Supported Models"="", "Instrument Options"="", "Check Status Callback"="", "Flags"=0, "Help"="Returns RB power values (power spectral density) for all measured list mode segments.\n\nAvailable Repeated Capabilities:\ninstance: i0, i1, i2, i3, i4, i5, i6, i7, i8, i9, i10, i11, i12, i13, i14, i15, i16, i17, i18, i19, i20, i21, i22, i23, i24, i25, i26, i27, i28, i29, i30, i31, i32\r\n\nRemote-control command(s):\nFETCh:NRMMw:MEAS<i>:MEValuation:LIST:MODulation:PSD:SDEViation?"}, {"Level"=5, "Class Only"=FALSE, "Identifier"="RSCMXPNRFR2M_ATTR_QUERY_MULTI_EVAL_MEASUREMENT_LIST_POWER_SPECTRAL_DENSITY_AVERAGE_LIMIT_CHECK_RESULTS", "Descriptive Name"="Query Multi Eval Measurement List Power Spectral Density Average Limit Check Results", "Data Type"=enum."RawString", "Command"="CALC:NRMM:MEAS{instance}:MEV:LIST:MOD:PSD:AVER?", "Access"=enum."Read Only", "Range Table"="", "Read Callback"="", "Write Callback"="", "Range Callback"="", "Check Callback"="", "Rngtable Callback"="", "Coerce Callback"="", "Supported Models"="", "Instrument Options"="", "Check Status Callback"="", "Flags"=0, "Help"="Returns the limit check results for the RB power values (power spectral density) for all measured list mode segments.\n\nAvailable Repeated Capabilities:\ninstance: i0, i1, i2, i3, i4, i5, i6, i7, i8, i9, i10, i11, i12, i13, i14, i15, i16, i17, i18, i19, i20, i21, i22, i23, i24, i25, i26, i27, i28, i29, i30, i31, i32\r\n\nRemote-control command(s):\nCALCulate:NRMMw:MEAS<i>:MEValuation:LIST:MODulation:PSD:AVERage?"}, {"Level"=5, "Class Only"=FALSE, "Identifier"="RSCMXPNRFR2M_ATTR_QUERY_MULTI_EVAL_MEASUREMENT_LIST_POWER_SPECTRAL_DENSITY_CURRENT_LIMIT_CHECK_RESULTS", "Descriptive Name"="Query Multi Eval Measurement List Power Spectral Density Current Limit Check Results", "Data Type"=enum."RawString", "Command"="CALC:NRMM:MEAS{instance}:MEV:LIST:MOD:PSD:CURR?", "Access"=enum."Read Only", "Range Table"="", "Read Callback"="", "Write Callback"="", "Range Callback"="", "Check Callback"="", "Rngtable Callback"="", "Coerce Callback"="", "Supported Models"="", "Instrument Options"="", "Check Status Callback"="", "Flags"=0, "Help"="Returns the limit check results for the RB power values (power spectral density) for all measured list mode segments.\n\nAvailable Repeated Capabilities:\ninstance: i0, i1, i2, i3, i4, i5, i6, i7, i8, i9, i10, i11, i12, i13, i14, i15, i16, i17, i18, i19, i20, i21, i22, i23, i24, i25, i26, i27, i28, i29, i30, i31, i32\r\n\nRemote-control command(s):\nCALCulate:NRMMw:MEAS<i>:MEValuation:LIST:MODulation:PSD:CURRent?"}, {"Level"=5, "Class Only"=FALSE, "Identifier"="RSCMXPNRFR2M_ATTR_QUERY_MULTI_EVAL_MEASUREMENT_LIST_POWER_SPECTRAL_DENSITY_MAXIMUM_LIMIT_CHECK_RESULTS", "Descriptive Name"="Query Multi Eval Measurement List Power Spectral Density Maximum Limit Check Results", "Data Type"=enum."RawString", "Command"="CALC:NRMM:MEAS{instance}:MEV:LIST:MOD:PSD:MAX?", "Access"=enum."Read Only", "Range Table"="", "Read Callback"="", "Write Callback"="", "Range Callback"="", "Check Callback"="", "Rngtable Callback"="", "Coerce Callback"="", "Supported Models"="", "Instrument Options"="", "Check Status Callback"="", "Flags"=0, "Help"="Returns the limit check results for the RB power values (power spectral density) for all measured list mode segments.\n\nAvailable Repeated Capabilities:\ninstance: i0, i1, i2, i3, i4, i5, i6, i7, i8, i9, i10, i11, i12, i13, i14, i15, i16, i17, i18, i19, i20, i21, i22, i23, i24, i25, i26, i27, i28, i29, i30, i31, i32\r\n\nRemote-control command(s):\nCALCulate:NRMMw:MEAS<i>:MEValuation:LIST:MODulation:PSD:MAXimum?"}, {"Level"=5, "Class Only"=FALSE, "Identifier"="RSCMXPNRFR2M_ATTR_QUERY_MULTI_EVAL_MEASUREMENT_LIST_POWER_SPECTRAL_DENSITY_MINIMUM_LIMIT_CHECK_RESULTS", "Descriptive Name"="Query Multi Eval Measurement List Power Spectral Density Minimum Limit Check Results", "Data Type"=enum."RawString", "Command"="CALC:NRMM:MEAS{instance}:MEV:LIST:MOD:PSD:MIN?", "Access"=enum."Read Only", "Range Table"="", "Read Callback"="", "Write Callback"="", "Range Callback"="", "Check Callback"="", "Rngtable Callback"="", "Coerce Callback"="", "Supported Models"="", "Instrument Options"="", "Check Status Callback"="", "Flags"=0, "Help"="Returns the limit check results for the RB power values (power spectral density) for all measured list mode segments.\n\nAvailable Repeated Capabilities:\ninstance: i0, i1, i2, i3, i4, i5, i6, i7, i8, i9, i10, i11, i12, i13, i14, i15, i16, i17, i18, i19, i20, i21, i22, i23, i24, i25, i26, i27, i28, i29, i30, i31, i32\r\n\nRemote-control command(s):\nCALCulate:NRMMw:MEAS<i>:MEValuation:LIST:MODulation:PSD:MINimum?"}, {"Level"=4, "Class Only"=TRUE, "Identifier"="", "Descriptive Name"="Transmit Time Error", "Data Type"=enum."ViInt32", "Command"="", "Access"=enum."Read Only", "Range Table"="", "Read Callback"="", "Write Callback"="", "Range Callback"="", "Check Callback"="", "Rngtable Callback"="", "Coerce Callback"="", "Supported Models"="", "Instrument Options"="", "Check Status Callback"="", "Flags"=0, "Help"="The following attributes return transmit time error values for all measured list mode segments."}, {"Level"=5, "Class Only"=FALSE, "Identifier"="RSCMXPNRFR2M_ATTR_FETCH_MULTI_EVAL_MEASUREMENT_LIST_TERR_AVERAGE_RESULTS", "Descriptive Name"="Fetch Multi Eval Measurement List TERR Average Results", "Data Type"=enum."RawString", "Command"="FETC:NRMM:MEAS{instance}:MEV:LIST:MOD:TERR:AVER?", "Access"=enum."Read Only", "Range Table"="", "Read Callback"="", "Write Callback"="", "Range Callback"="", "Check Callback"="", "Rngtable Callback"="", "Coerce Callback"="", "Supported Models"="", "Instrument Options"="", "Check Status Callback"="", "Flags"=0, "Help"="Returns transmit time error values for all measured list mode segments.\n\nAvailable Repeated Capabilities:\ninstance: i0, i1, i2, i3, i4, i5, i6, i7, i8, i9, i10, i11, i12, i13, i14, i15, i16, i17, i18, i19, i20, i21, i22, i23, i24, i25, i26, i27, i28, i29, i30, i31, i32\r\n\nRemote-control command(s):\nFETCh:NRMMw:MEAS<i>:MEValuation:LIST:MODulation:TERRor:AVERage?"}, {"Level"=5, "Class Only"=FALSE, "Identifier"="RSCMXPNRFR2M_ATTR_FETCH_MULTI_EVAL_MEASUREMENT_LIST_TERR_CURRENT_RESULTS", "Descriptive Name"="Fetch Multi Eval Measurement List TERR Current Results", "Data Type"=enum."RawString", "Command"="FETC:NRMM:MEAS{instance}:MEV:LIST:MOD:TERR:CURR?", "Access"=enum."Read Only", "Range Table"="", "Read Callback"="", "Write Callback"="", "Range Callback"="", "Check Callback"="", "Rngtable Callback"="", "Coerce Callback"="", "Supported Models"="", "Instrument Options"="", "Check Status Callback"="", "Flags"=0, "Help"="Returns transmit time error values for all measured list mode segments.\n\nAvailable Repeated Capabilities:\ninstance: i0, i1, i2, i3, i4, i5, i6, i7, i8, i9, i10, i11, i12, i13, i14, i15, i16, i17, i18, i19, i20, i21, i22, i23, i24, i25, i26, i27, i28, i29, i30, i31, i32\r\n\nRemote-control command(s):\nFETCh:NRMMw:MEAS<i>:MEValuation:LIST:MODulation:TERRor:CURRent?"}, {"Level"=5, "Class Only"=FALSE, "Identifier"="RSCMXPNRFR2M_ATTR_FETCH_MULTI_EVAL_MEASUREMENT_LIST_TERR_EXTREME_RESULTS", "Descriptive Name"="Fetch Multi Eval Measurement List TERR Extreme Results", "Data Type"=enum."RawString", "Command"="FETC:NRMM:MEAS{instance}:MEV:LIST:MOD:TERR:EXTR?", "Access"=enum."Read Only", "Range Table"="", "Read Callback"="", "Write Callback"="", "Range Callback"="", "Check Callback"="", "Rngtable Callback"="", "Coerce Callback"="", "Supported Models"="", "Instrument Options"="", "Check Status Callback"="", "Flags"=0, "Help"="Returns transmit time error values for all measured list mode segments.\n\nAvailable Repeated Capabilities:\ninstance: i0, i1, i2, i3, i4, i5, i6, i7, i8, i9, i10, i11, i12, i13, i14, i15, i16, i17, i18, i19, i20, i21, i22, i23, i24, i25, i26, i27, i28, i29, i30, i31, i32\r\n\nRemote-control command(s):\nFETCh:NRMMw:MEAS<i>:MEValuation:LIST:MODulation:TERRor:EXTReme?"}, {"Level"=5, "Class Only"=FALSE, "Identifier"="RSCMXPNRFR2M_ATTR_QUERY_MULTI_EVAL_MEASUREMENT_LIST_TERR_AVERAGE_LIMIT_CHECK_RESULTS", "Descriptive Name"="Query Multi Eval Measurement List TERR Average Limit Check Results", "Data Type"=enum."RawString", "Command"="CALC:NRMM:MEAS{instance}:MEV:LIST:MOD:TERR:AVER?", "Access"=enum."Read Only", "Range Table"="", "Read Callback"="", "Write Callback"="", "Range Callback"="", "Check Callback"="", "Rngtable Callback"="", "Coerce Callback"="", "Supported Models"="", "Instrument Options"="", "Check Status Callback"="", "Flags"=0, "Help"="Returns the limit check results for the transmit time error values for all measured list mode segments.\n\nAvailable Repeated Capabilities:\ninstance: i0, i1, i2, i3, i4, i5, i6, i7, i8, i9, i10, i11, i12, i13, i14, i15, i16, i17, i18, i19, i20, i21, i22, i23, i24, i25, i26, i27, i28, i29, i30, i31, i32\r\n\nRemote-control command(s):\nCALCulate:NRMMw:MEAS<i>:MEValuation:LIST:MODulation:TERRor:AVERage?"}, {"Level"=5, "Class Only"=FALSE, "Identifier"="RSCMXPNRFR2M_ATTR_QUERY_MULTI_EVAL_MEASUREMENT_LIST_TERR_CURRENT_LIMIT_CHECK_RESULTS", "Descriptive Name"="Query Multi Eval Measurement List TERR Current Limit Check Results", "Data Type"=enum."RawString", "Command"="CALC:NRMM:MEAS{instance}:MEV:LIST:MOD:TERR:CURR?", "Access"=enum."Read Only", "Range Table"="", "Read Callback"="", "Write Callback"="", "Range Callback"="", "Check Callback"="", "Rngtable Callback"="", "Coerce Callback"="", "Supported Models"="", "Instrument Options"="", "Check Status Callback"="", "Flags"=0, "Help"="Returns the limit check results for the transmit time error values for all measured list mode segments.\n\nAvailable Repeated Capabilities:\ninstance: i0, i1, i2, i3, i4, i5, i6, i7, i8, i9, i10, i11, i12, i13, i14, i15, i16, i17, i18, i19, i20, i21, i22, i23, i24, i25, i26, i27, i28, i29, i30, i31, i32\r\n\nRemote-control command(s):\nCALCulate:NRMMw:MEAS<i>:MEValuation:LIST:MODulation:TERRor:CURRent?"}, 
